vi "Count Up (U16).vi"(7 "reset":bool, 11 "increment":bool) -> (3 "count out":u16)   [LabVIEW 2023, in "CHDR Support.lvlib"]
doc: "16-bit counter that can increment when reset is true."
uses:
  CHDR Support.lvlib
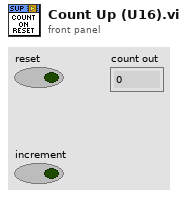
[diagram p1: front panel]
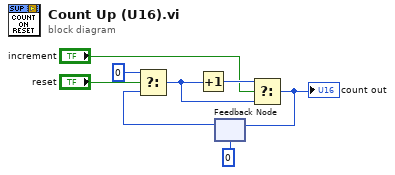
[diagram p0: block diagram]
diagram:
  n1 = feedback #1(u16 0 ("count in")) -> (w7:u16)
  n2 = Select(t=u16 0 ("count in"), s="reset", f=w7) -> (s? t:f=w8:u16)
  n3 = Increment(x=w8) -> (x+1=w4:u16)
  n4 = Select(t=w4, s="increment", f=w8) -> (s? t:f=w6:u16)
  "count out" <- w6
  n5 = feedback-in #1(w6) -> ()
